vi "Spartan HTTP Create Session.vi"(4 "error in (no error)":errorcluster, 5 "remote port":u16, 6 "address":string, 7 "id":refnum<k5>) -> (0 "error out":errorcluster, 2 "num requests":u32, 3 "HTTP Data":T1 {"object data"."time" format="%0.2f"})   [LabVIEW 2011]
doc: "Creates a unique object that has to be destroyed with Object Destroy."
uses:
  Spartan HTTP Session.ctl
  ITK EXT/http/http_obj.llb/HTTP Session Data.ctl
  ITK EXT/utils/keyedarr.llb/Keyed Array.ctl
  Spartan HTTP Server Globals.vi
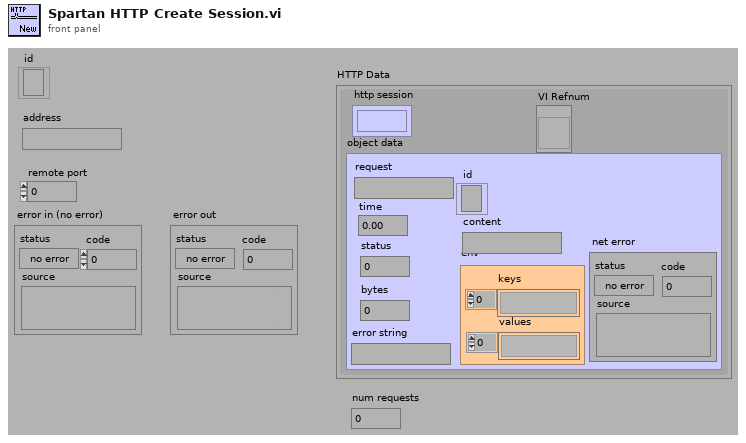
[diagram p1: front panel]
types:
  T1 = typedef "Spartan HTTP Session.ctl" = cluster{"http session":refnum<k1>, "object data":T2, "VI Refnum":refnum<vi>}
  T2 = typedef "HTTP Session Data.ctl" = cluster{"request":string, "time":dbl, "status":i32, "error string":string, "bytes":i32, "env":T3, "content":string, "id":refnum<k5>, "net error":errorcluster}
  T3 = typedef "Keyed Array.ctl" = cluster{"keys":string[], "values":string[]}
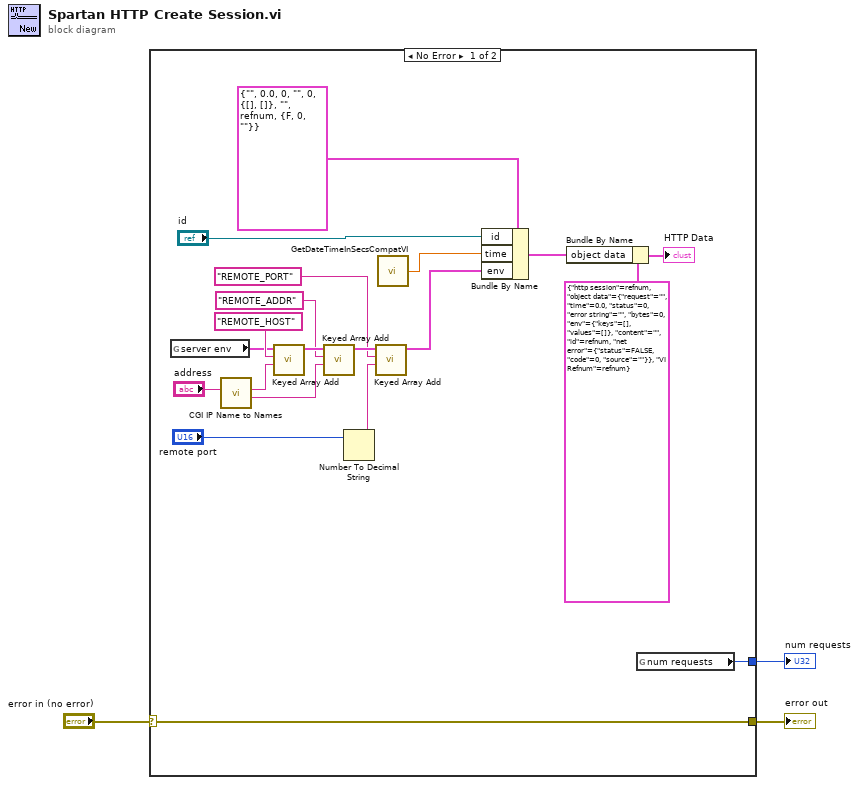
[diagram p0: block diagram]
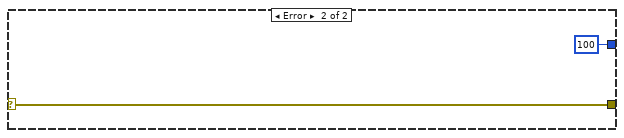
[diagram p2: hidden frame]
diagram:
  n1 = case shown="No Error" "error in (no error)" {
    selector: "error in (no error)" -> [w5 w25]
    tunnel: [w5 w25] -> w3
    tunnel: [w4 u32 100] -> w1
    frame No Error {
      n2 = global read "Spartan HTTP Server Globals.vi" "server env"() -> (w15:T3)
      n3 = call "CGI IP Name to Names.vi"("name"="address") -> ("dot name"=w18:string, "domain name"=w19:string)  [unwired: 1 in, 4 out]
      n4 = call "Keyed Array Add.vi"("value"=w19, "key"="REMOTE_HOST", "array in"=w15) -> ("array out"=w20:T3)  [unwired: 1 in, 3 out]
      n5 = call "Keyed Array Add.vi"("value"=w18, "key"="REMOTE_ADDR", "array in"=w20) -> ("array out"=w14:T3)  [unwired: 1 in, 3 out]
      n6 = Number To Decimal String(number="remote port") -> (decimal integer string=w10:string)  [unwired: 1 out]
      n7 = call "Keyed Array Add.vi"("value"=w10, "key"="REMOTE_PORT", "array in"=w14) -> ("array out"=w13:T3)  [unwired: 1 in, 3 out]
      n8 = call <vilib>:"GetDateTimeInSecsCompatVI.vi"() -> ("double precision float"=w22:dbl)  [unwired: 1 out]
      n9 = Bundle By Name(cluster=T2 {"request"="", "time"=0.0, "status"=0, "error string"="", "bytes"=0, "env"={"keys"=[], "values"=[]}, "content"="", "id"=refnum, "net error"={"status"=FALSE, "code"=0, "source"=""}} ("object data"), "id"="id", "time"=w22, "env"=w13) -> (w7:T2)
      n10 = Bundle By Name(cluster=T1 {"http session"=refnum, "object data"={"request"="", "time"=0.0, "status"=0, "error string"="", "bytes"=0, "env"={"keys"=[], "values"=[]}, "content"="", "id"=refnum, "net error"={"status"=FALSE, "code"=0, "source"=""}}, "VI Refnum"=refnum} ("empty object"), "object data"=w7) -> (→"HTTP Data":T1)
      n11 = global read "Spartan HTTP Server Globals.vi" "num requests"() -> (w4:u32)
    }
    frame Error {
    }
  }
  "error out" <- w3
  "num requests" <- w1
